vi "Set Condition for Waveform Stream (All Data).vi"(8 "error in (no error)":errorcluster, 11 "WaveformStreamSpecification in":T1) -> (0 "error out":errorcluster, 3 "WaveformStreamSpecification out":T1)   [LabVIEW 2020, in "NI_VS Waveform Streaming Interface.lvlib"]
doc: "Defines the condition under which NI VeriStand streams waveform data to a host computer."
uses:
  <vilib>/NI VeriStand/Execution/WaveformStreaming/NI_VS Waveform Streaming Interface.lvlib
  <vilib>/NI VeriStand/Execution/WaveformStreaming/WaveformStreamSpecification.ctl
  NationalInstruments.VeriStand.ClientAPI
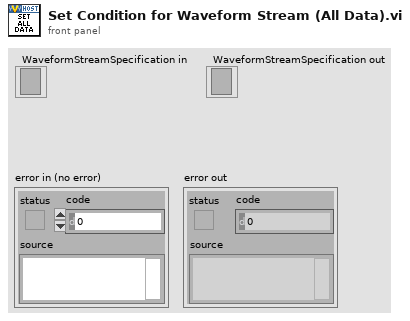
[diagram p1: front panel]
types:
  T1 = typedef "NI_VS Waveform Streaming Interface.lvlib/WaveformStreamSpecification.ctl" = refnum<k24>
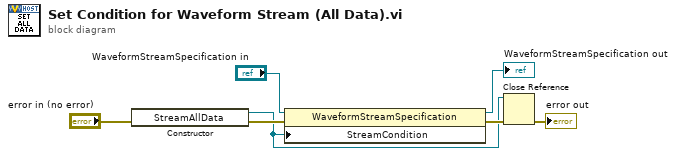
[diagram p0: block diagram]
diagram:
  n1 = constructor class="StreamAllData"(error in="error in (no error)") -> (reference out=w2:refnum<k24>, error out=w4:errorcluster)  [unwired: 2 in, 1 out]
  n2 = property class="WaveformStreamSpecification"(reference="WaveformStreamSpecification in", error in=w4, "StreamCondition"=w2) -> (reference out=→"WaveformStreamSpecification out":T1, error out=w3:errorcluster)
  n3 = Close Reference(reference=w2, error in (no error)=w3) -> (error out=→"error out":errorcluster)
